vi "DBFL1dll.vi"(8 "error in (no error)":errorcluster, 11 "Inputs":T2) -> (0 "error out":errorcluster, 3 "Outputs":T1)   [LabVIEW 2016]
doc: "SINGLE-PHASE FLASH SUBROUTINES\n\nsubroutine DBFL1dll(d, b, z, ab, t, p, ierr, herr, ab_length, herr_length)\n\nGeneral single-phase calculation given density, composition, and either pressure, energy, enthalpy, or entropy.\nThe character string ab specifies the inputs. This routine should ONLY be called by ABFL1.\n\nINPUTS:\nd -- Molar density [mol/L]\nb -- Second property (pressure, energy, enthalpy, or entropy)\nz -- Composition (array of mole fractions)\nab -- Character*2 string defining the inputs: ‘DH’, ‘DS’, ‘DE’, or ‘DP’\n\nOUTPUTS:\nt -- Temperature [K]\np -- Pressure [kPa]\nierr -- Error flag: 0 = Successful, 207 = Density or pressure equal to zero, no solution available, 208= Iteration did not converge\nherr -- Error string (character*255 variable if ierr<>0)\nab_length -- length of variable ab (default: 2)\nherr_length -- length of variable herr (default: 255)"
uses:
  REFPROP.DLL
panel:
  # "REFPROP-DBFL1dll.vi"
  # "void  DBFL1dll(double *d, double *b, double *z, CStr ab, double *t, double *p, int32_t *ierr, CStr herr, int32_t ab_length, int32_t herr_length)"
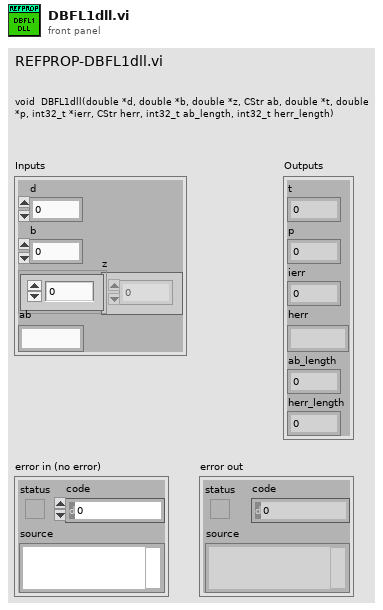
[diagram p1: front panel]
types:
  T1 = cluster{"t":dbl, "p":dbl, "ierr":i32, "herr":string, "ab_length":i32, "herr_length":i32}
  T2 = cluster{"d":dbl, "b":dbl, "z":dbl[], "ab":string}
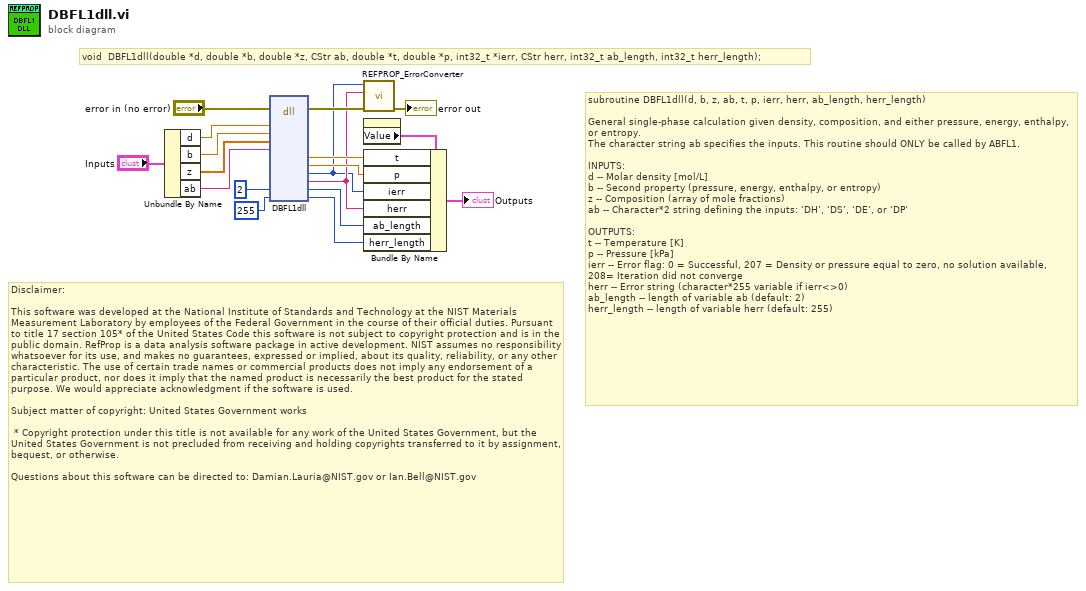
[diagram p0: block diagram]
diagram:
  # "Disclaimer:\n\nThis software was developed at the National Institute of Standards and Technology at the NIST Materials Measurement Laboratory by employees of the Federal Government in the course of their official duties. Pursuant to title 17 section 105* of the United States Code this software is not subject to copyright protection and is in the public domain. RefProp is a data analysis software package in active development. NIST assumes no responsibility whatsoever for its use, and makes no guarantees, expressed or implied, about its quality, reliability, or any other characteristic. The use of certain trade names or commercial products does not imply any endorsement of a particular product, nor does it imply that the named product is necessarily the best product for the stated purpose. We would appreciate acknowledgment if the software is used.\n \nSubject matter of copyright: United States Government works\n  \n * Copyright protection under this title is not available for any work of the United States Government, but the United States Government is not precluded from receiving and holding copyrights transferred to it by assignment, bequest, or otherwise.\n\nQuestions about this software can be directed to: Damian.Lauria@NIST.gov or Ian.Bell@NIST.gov"
  # "void  DBFL1dll(double *d, double *b, double *z, CStr ab, double *t, double *p, int32_t *ierr, CStr herr, int32_t ab_length, int32_t herr_length);"
  # "subroutine DBFL1dll(d, b, z, ab, t, p, ierr, herr, ab_length, herr_length)\n\nGeneral single-phase calculation given density, composition, and either pressure, energy, enthalpy, or entropy.\nThe character string ab specifies the inputs. This routine should ONLY be called by ABFL1.\n\nINPUTS:\nd -- Molar density [mol/L]\nb -- Second property (pressure, energy, enthalpy, or entropy)\nz -- Composition (array of mole fractions)\nab -- Character*2 string defining the inputs: ‘DH’, ‘DS’, ‘DE’, or ‘DP’\n\nOUTPUTS:\nt -- Temperature [K]\np -- Pressure [kPa]\nierr -- Error flag: 0 = Successful, 207 = Density or pressure equal to zero, no solution available, 208= Iteration did not converge\nherr -- Error string (character*255 variable if ierr<>0)\nab_length -- length of variable ab (default: 2)\nherr_length -- length of variable herr (default: 255)"
  n1 = Unbundle By Name("Inputs") -> ("d"=w9:dbl, "b"=w10:dbl, "z"=w11:dbl[], "ab"=w12:string)
  n2 = dll-call lib="S:/009 - Testing/02 - Performance Testing/REFPROP/REFPROP.*" fn="DBFL1dll"(error in="error in (no error)", "d"=w9, "b"=w10, "z"=w11, "ab"=w12, "ab_length"=2, "herr_length"=255 ("ln2")) -> (error out=w17:errorcluster, "t"=w4:dbl, "p"=w5:dbl, "ierr"=w1:i32, "herr"=w2:string, "ab_length"=w6:i32, "herr_length"=w7:i32)  [unwired: 11 in, 1 out]
  n3 = call "REFPROP_ErrorConverter.vi"("error in (no error)"=w17, "Error Message"=w2, "Error Code"=w1) -> ("error out"=→"error out":errorcluster)  [unwired: 8 in]
  n4 = property on="Outputs" class="Clust (strict)"() -> ("Value"=w8:T1)  [unwired: 2 in, 2 out]
  n5 = Bundle By Name(cluster=w8, "t"=w4, "p"=w5, "ierr"=w1, "herr"=w2, "ab_length"=w6, "herr_length"=w7) -> (→"Outputs":T1)
